vi "Generate and Acquire Waveform.vi"() -> ()   [LabVIEW 2010]
doc: "This example shows how to acquire 16k samples of continuous signal on fast analog inputs. Signal will be acquired simultaneously with generated signal. Time length of the acquired signal depends on the time scale of a buffer that can be set with a decimation factor. Decimations and time scales of a buffer are given in the table below. Voltage range of fast analog inputs on the Red Pitaya depends on gain setting that can be set by jumpers. HV setting is for input range to ±20V, while LV sets input range to ±1V."
uses:
  RedPitaya.lvlib
panel:
  in  "Trigger Mode":string(combo)="CH1_PE"
  in  "Trigger Level (0 mV)":i32=100
  in  "Delay (# Samples)":i32
  in  "Averaging":enum16{"None", "AVG ON", "AVG OFF"}(ring)
  in  "Duty Cycle":i32=-1 min=-1 max=100
  in  "Phase":i32=361
  in  "DC Offset":dbl=2.0
  in  "Amplitude":dbl=2.0
  in  "Decimation":u32(ring)=8 items=["65536"=65536, "8192"=8192, "1024"=1024, "64"=64, "8"=8, "1"=1]
  in  "Channel (1|2)":u16(ring)=1 items=["Channel 1"=1, "Channel 2"=2]
  in  "Waveform Function":u16(ring)=1 items=["", "Sine", "Square", "Triangle", "Sawtooth UP", "Sawtooth Down", "PWM"]
  in  "Frequency (1000 Hz)":i32=10000
  out "Waveform Graph":dbl[](graph)
  in  "IP address":string="192.168.1.100"
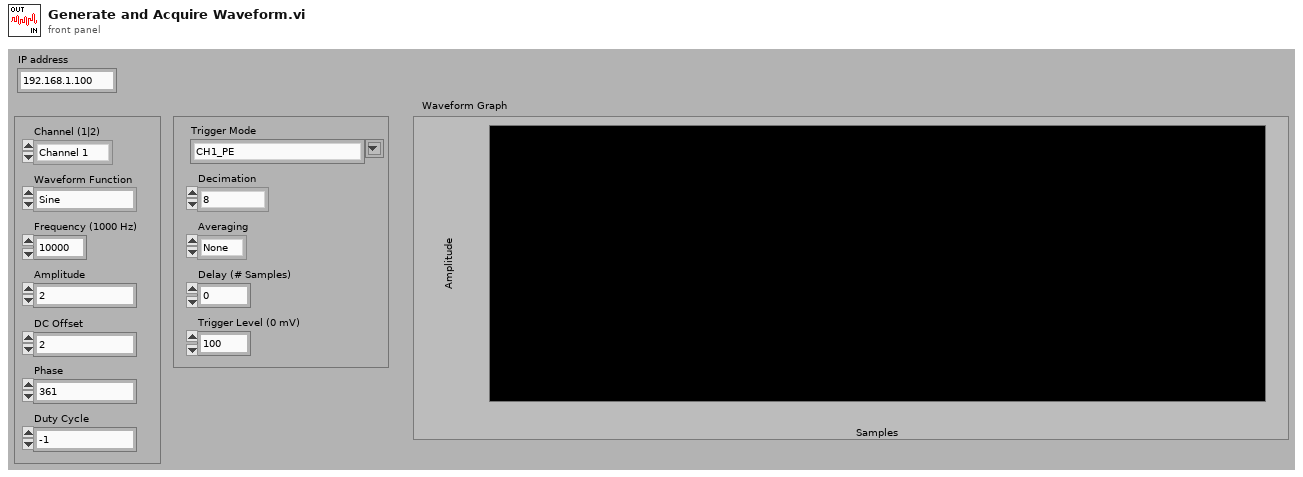
[diagram p1: front panel]
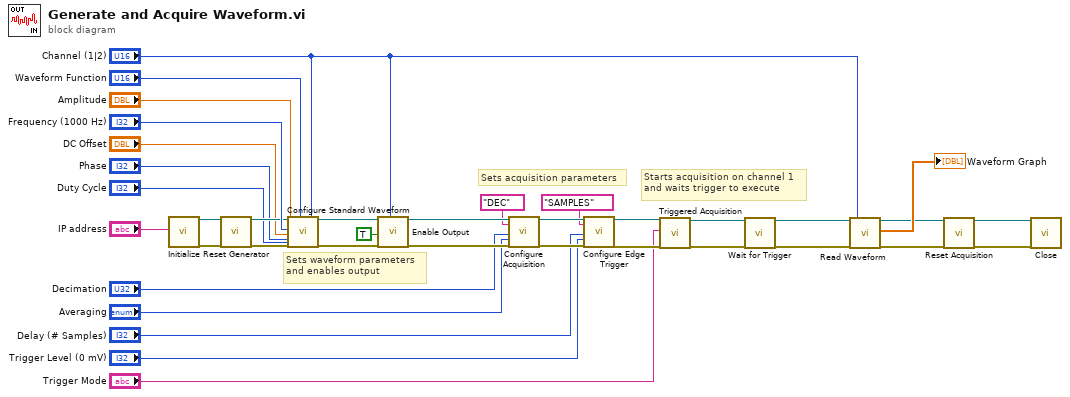
[diagram p0: block diagram]
diagram:
  # "Starts acquisition on channel 1\nand waits trigger to execute"
  # "Sets acquisition parameters"
  # "Sets waveform parameters\nand enables output"
  n1 = call "Initialize.vi"("IP address"="IP address") -> ("RedPitaya TCP Connection"=w12:refnum<k5>, "error out"=w10:errorcluster)  [unwired: 17 in]
  n2 = call "Reset Generator.vi"("RedPitaya connection in"=w12, "error in"=w10) -> ("RedPitaya connection out"=w11:refnum<k5>, "error out"=w9:errorcluster)  [unwired: 16 in]
  n3 = call "Configure Standard Waveform.vi"("RedPitaya connection in"=w11, "Amplitude"="Amplitude", "Frequency"="Frequency (1000 Hz)", "DC Offset"="DC Offset", "Phase"="Phase", "error in"=w9, "Channel #"="Channel (1|2)", "Duty Cycle"="Duty Cycle", "Waveform Function"="Waveform Function") -> ("RedPitaya connection out"=w33:refnum<k5>, "error out"=w32:errorcluster)  [unwired: 9 in]
  n4 = call "Enable Output.vi"("RedPitaya connection in"=w33, "Generation (T: Enable)"=TRUE, "error in"=w32, "Channel #"="Channel (1|2)") -> ("RedPitaya connection out"=w30:refnum<k5>, "error out"=w29:errorcluster)  [unwired: 14 in]
  n5 = call "Configure Acquisition.vi"("RedPitaya connection in"=w30, "Decimation/Sampling Rate"="DEC", "Decimation"="Decimation", "Averaging"="Averaging", "error in"=w29) -> ("RedPitaya connection out"=w27:refnum<k5>, "error out"=w26:errorcluster)  [unwired: 13 in]
  n6 = call "Configure Edge Trigger.vi"("RedPitaya connection in"=w27, "Trigger Delay mode"="SAMPLES", "Delay (# Samples)"="Delay (# Samples)", "Trigger Level (0 mV)"="Trigger Level (0 mV)", "error in"=w26) -> ("RedPitaya connection out"=w36:refnum<k5>, "error out"=w35:errorcluster)  [unwired: 13 in]
  n7 = call "Triggered Acquisition.vi"("RedPitaya TCP connection in"=w36, "Trigger Mode"="Trigger Mode", "error in"=w35) -> ("RedPitaya TCP connection out"=w24:refnum<k5>, "error out"=w21:errorcluster)  [unwired: 15 in]
  n8 = call "Wait for Trigger.vi"("RedPitaya TCP connection in"=w24, "error in"=w21) -> ("RedPitaya TCP connection out"=w23:refnum<k5>, "error out"=w22:errorcluster)  [unwired: 16 in]
  n9 = call "Read Waveform.vi"("RedPitaya TCP Connection in"=w23, "error in"=w22, "Channel #"="Channel (1|2)") -> ("RedPitaya TCP Connection out"=w20:refnum<k5>, "Measurement Array"=→"Waveform Graph":dbl[], "error out"=w18:errorcluster)  [unwired: 14 in]
  n10 = call "Reset Acquisition.vi"("RedPitaya connection in"=w20, "error in"=w18) -> ("RedPitaya connection out"=w19:refnum<k5>, "error out"=w17:errorcluster)  [unwired: 16 in]
  n11 = call "Close.vi"("connection ID"=w19, "error in"=w17) -> ()  [unwired: 17 in, 1 out]
